vi "CRYCalc Result mean and abs standard.vi"(7 "Step Setup VI No":i32, 8 "Statistic Run Number":i32, 9 "Work in":u16, 11 "Results in":T2 {"Margin" format="%.2f"}) -> (0 "Boolean":bool, 1 "Margin Std Dev Out":T1[](array[typedef]) {"Z data" items=["dB", "Lin"]; "X data" items=["dB", "Lin"]; "Y data" items=["dB", "Lin"]; "Z dB ref" format="%.1f"; "Z axis" items=["Log", "Lin"]; "X dB ref" format="%.1f"; "X axis" items=["Log", "Lin"]; "Y axis" items=["Log", "Lin"]; "Y dB ref" format="%.1f"; "Curve"."z" format="%.2f"; "Curve"."y" format="%.2f"; "Curve"."x" format="%.2f"}, 3 "Margin mean Out":T1[](array[typedef]) {"Z data" items=["dB", "Lin"]; "X data" items=["dB", "Lin"]; "Y data" items=["dB", "Lin"]; "Z dB ref" format="%.1f"; "Z axis" items=["Log", "Lin"]; "X dB ref" format="%.1f"; "X axis" items=["Log", "Lin"]; "Y axis" items=["Log", "Lin"]; "Y dB ref" format="%.1f"; "Curve"."z" format="%.2f"; "Curve"."y" format="%.2f"; "Curve"."x" format="%.2f"})   [LabVIEW 2013]
uses:
  Typedef Control/CRYResult Cluster Array.ctl
  Typedef Control/CRYResult Cluster.ctl
  Typedef Control/CRYData Cluster.ctl
  CRYStatistics Global.vi
  <vilib>/Analysis/NI_AALBase.lvlib
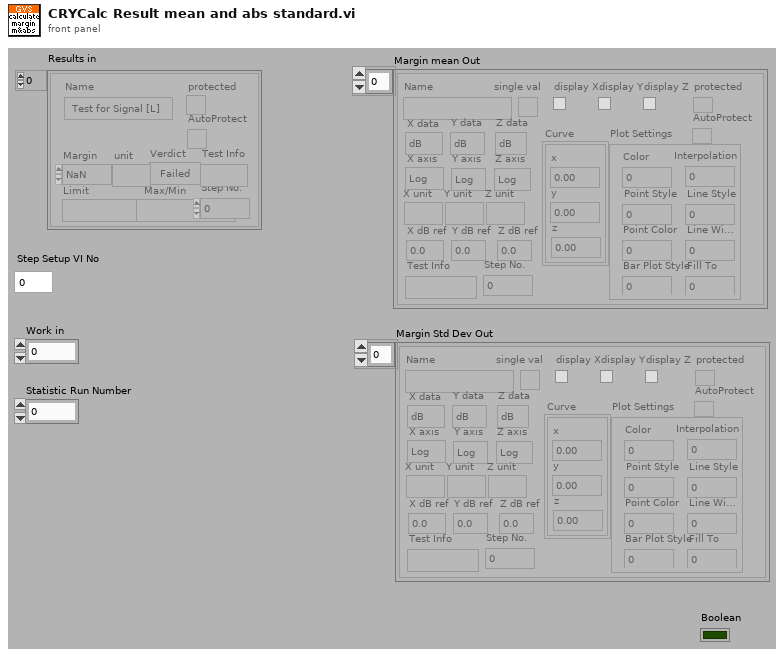
[diagram p1: front panel]
types:
  T1 = typedef "CRYData Cluster.ctl" = cluster{"Name":string, "Curve":cluster{"x":dbl, "y":dbl, "z":dbl}[], "X data":u16, "Y data":u16, "Z data":u16, "X axis":u16, "Y axis":u16, "Z axis":u16, "X unit":string, "Y unit":string, "Z unit":string, "X dB ref":dbl, "Y dB ref":dbl, "Z dB ref":dbl, "single val":bool, "protected":bool, "display X":bool, "display Y":bool, "display Z":bool, "Test Info":string, "Step No.":i32, "Plot Settings":cluster{"Color":u32, "Interpolation":u8, "Point Style":u8, "Line Style":u8, "Point Color":u32, "Line Width":u8, "Bar Plot Style":u8, "Fill To":i16}, "AutoProtect":bool}
  T2 = typedef "CRYResult Cluster Array.ctl" = T3[]
  T3 = typedef "CRYResult Cluster.ctl" = cluster{"Name":string, "Margin":dbl, "unit":string, "Verdict":bool, "Limit":string, "Max/Min":string, "protected":bool, "Step No.":i32, "Test Info":string, "AutoProtect":bool}
  T4 = enum32{"English", "Chinese", "Korean", "Japanese", "Russian", "Chinese traditional"}
  T5 = typedef "CRYData Cluster Array.ctl" = T1[]
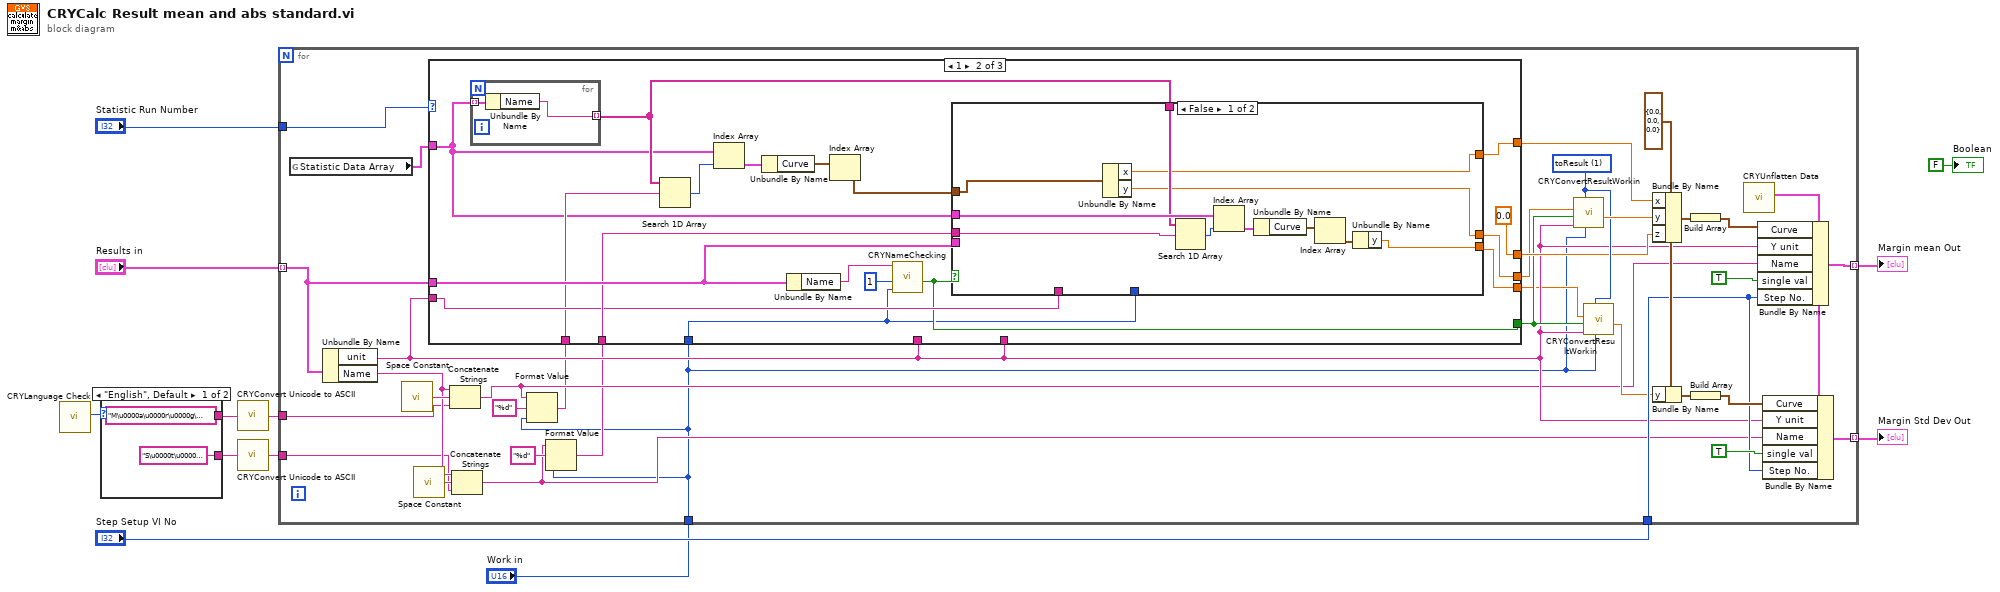
[diagram p0: block diagram]
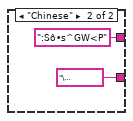
[diagram p2: hidden frame]
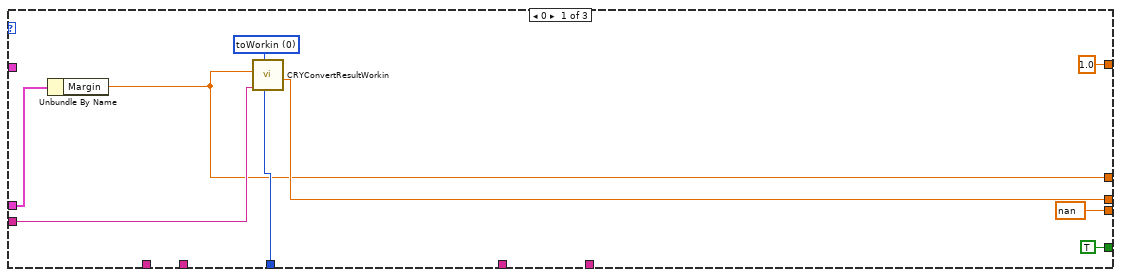
[diagram p3: hidden frame]
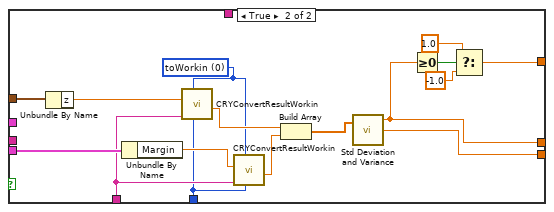
[diagram p4: hidden frame]
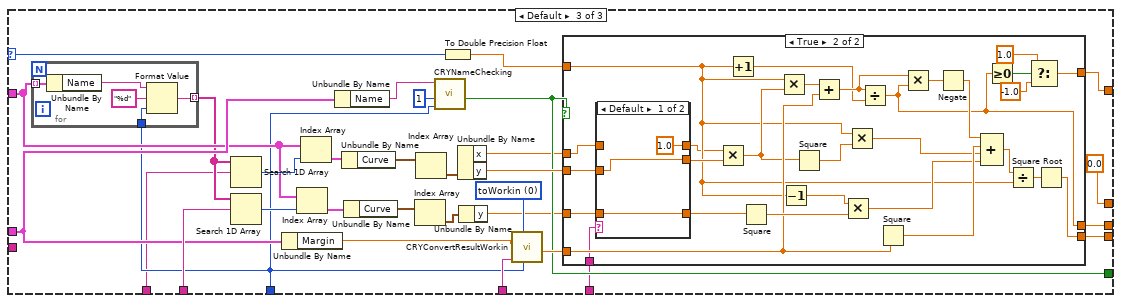
[diagram p5: hidden frame]
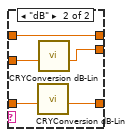
[diagram p7: hidden frame]
diagram:
  n1 = call "CRYLanguage Check.vi"() -> ("Language"=w5:T4)  [unwired: 10 in, 1 out]
  n2 = case shown="\"English\", Default" w5 {
    tunnel: ["M\u0000a\u0000r\u0000g\u0000i\u0000n\u0000 \u0000M\u0000e\u0000a\u0000n\u0000" ("format string") ":Sô•s^GW<P" ("format string")] -> w6
    tunnel: ["S\u0000t\u0000d\u0000 \u0000D\u0000e\u0000v\u0000" ("format string") "\u0007hÆQî]" ("format string")] -> w4
    frame "English", Default {
    }
    frame "Chinese" {
    }
  }
  n3 = call "CRYConvert Unicode to ASCII.vi"("Unicode"=w6) -> ("ASCII"=w3:string)  [unwired: 4 in]
  n4 = call "CRYConvert Unicode to ASCII.vi"("Unicode"=w4) -> ("ASCII"=w2:string)  [unwired: 4 in]
  n5 = for {
    tunnel: "Results in" -> [w33] mode=indexing
    tunnel: [w48] -> w11 mode=indexing
    tunnel: [w42] -> w10 mode=indexing
    tunnel: "Step Setup VI No" -> [w41]
    tunnel: "Statistic Run Number" -> [w40]
    tunnel: w3 -> [w35]
    tunnel: w2 -> [w34]
    tunnel: "Work in" -> [w17]
    w31 = u16 1 items=["toWorkin", "toResult"] ("Type")
    w43 = cluster{"x":dbl, "y":dbl, "z":dbl} {"x"=0.0, "y"=0.0, "z"=0.0}
    n6 = global read "CRYStatistics Global.vi" "Statistic Data Array"() -> (w36:T5)
    n7 = Unbundle By Name(w33) -> ("unit"=w27:string, "Name"=w37:string)
    n8 = call <vilib>:"Space Constant.vi"() -> ("String"=w39:string)
    n9 = call <vilib>:"Space Constant.vi"() -> ("String"=w38:string)
    n10 = Concatenate Strings(w37, w39, w35) -> (w22:string)
    n11 = Concatenate Strings(w37, w38, w34) -> (w19:string)
    n12 = Format Value(string ("")=w22, format string="%d", value (0)=w17) -> (output string=w21:string)
    n13 = Format Value(string ("")=w19, format string="%d", value (0)=w17) -> (output string=w18:string)
    n14 = case shown="1" w40 {
      selector: w40 -> [_ _ w117]
      tunnel: w33 -> [w59 w73 w124]
      tunnel: w18 -> [_ w70 w137]
      tunnel: [w57 w75 w129] -> w26
      tunnel: [nan ("y") w74 w128] -> w25
      tunnel: w36 -> [_ w62 w111]
      tunnel: w27 -> [w60 w69 _]
      tunnel: w17 -> [w55 w61 w109]
      tunnel: w27 -> [_ _ w123]
      tunnel: [w54 0.0 ("Margin") 0.0 ("Margin")] -> w29
      tunnel: [TRUE ("Out Calcurated") w66 w116] -> w28
      tunnel: w27 -> [_ _ w115]
      tunnel: [1.0 ("f") w65 w113] -> w24
      tunnel: w21 -> [_ w64 w108]
      frame 0 {
        w58 = u16 0 items=["toWorkin", "toResult"] ("Type")
        n15 = Unbundle By Name(w59) -> ("Margin"=w54:dbl)
        n16 = call "CRYConvertResultWorkin.vi"("Work in"=w55, "Type"=w58, "unit"=w60, "Margin In"=w54) -> ("Margin Out"=w57:dbl)  [unwired: 7 in]
      }
      frame 1 {
        n17 = for {
          tunnel: w62 -> [w80] mode=indexing
          tunnel: [w79] -> w63 mode=indexing
          n18 = Unbundle By Name(w80) -> ("Name"=w79:string)
        }
        n19 = Search 1D Array(1D array=w63, element=w64) -> (index of element=w78:i32)  [unwired: 1 in]
        n20 = Index Array(array=w62, index=w78) -> (element=w77:T1)
        n21 = Unbundle By Name(w77) -> ("Curve"=w76:cluster{"x":dbl, "y":dbl, "z":dbl}[])
        n22 = Unbundle By Name(w73) -> ("Name"=w72:string)
        n23 = Index Array(array=w76) -> (element=w67:cluster{"x":dbl, "y":dbl, "z":dbl})  [unwired: 1 in]
        n24 = call "CRYNameChecking.vi"("Curve Name"=w72, "Mode"=i8 1, "Work in"=w61) -> ("Out Calcurated"=w66:bool)  [unwired: 7 in]
        n25 = case shown="False" w66 {
          tunnel: w67 -> [w84 w99]
          tunnel: [w83 w94] -> w75
          tunnel: [w82 w92] -> w74
          tunnel: w73 -> [_ w106]
          tunnel: w70 -> [w87 _]
          tunnel: w62 -> [w86 _]
          tunnel: w63 -> [w85 _]
          tunnel: w69 -> [_ w103]
          tunnel: w61 -> [_ w102]
          tunnel: [w81 w93] -> w65
          frame False {
            n26 = Unbundle By Name(w84) -> ("x"=w81:dbl, "y"=w83:dbl)
            n27 = Search 1D Array(1D array=w85, element=w87) -> (index of element=w88:i32)  [unwired: 1 in]
            n28 = Index Array(array=w86, index=w88) -> (element=w89:T1)
            n29 = Unbundle By Name(w89) -> ("Curve"=w90:cluster{"x":dbl, "y":dbl, "z":dbl}[])
            n30 = Index Array(array=w90) -> (element=w91:cluster{"x":dbl, "y":dbl, "z":dbl})  [unwired: 1 in]
            n31 = Unbundle By Name(w91) -> ("y"=w82:dbl)
          }
          frame True {
            w101 = u16 0 items=["toWorkin", "toResult"] ("Type")
            n32 = Unbundle By Name(w99) -> ("z"=w98:dbl)
            n33 = Unbundle By Name(w106) -> ("Margin"=w104:dbl)
            n34 = call "CRYConvertResultWorkin.vi"("Work in"=w102, "Type"=w101, "unit"=w103, "Margin In"=w98) -> ("Margin Out"=w105:dbl)  [unwired: 7 in]
            n35 = call "CRYConvertResultWorkin.vi"("Work in"=w102, "Type"=w101, "unit"=w103, "Margin In"=w104) -> ("Margin Out"=w100:dbl)  [unwired: 7 in]
            n36 = Build Array(w105, w100) -> (w107:dbl[])
            n37 = call <vilib>:"Std Deviation and Variance.vi"("X"=w107) -> ("mean"=w94:dbl, "standard deviation"=w92:dbl)  [unwired: 1 in, 1 out]
            n38 = Greater Or Equal To 0?(x=w94) -> (x >= 0?=w95:bool)
            n39 = Select(t=1.0, s=w95, f=-1.0) -> (s? t:f=w93:dbl)
          }
        }
      }
      frame Default {
        w118 = u16 0 items=["toWorkin", "toResult"] ("Type")
        n40 = for {
          tunnel: w111 -> [w143] mode=indexing
          tunnel: w109 -> [w140]
          tunnel: [w139] -> w110 mode=indexing
          n41 = Unbundle By Name(w143) -> ("Name"=w141:string)
          n42 = Format Value(string ("")=w141, format string="%d", value (0)=w140) -> (output string=w139:string)
        }
        n43 = Search 1D Array(1D array=w110, element=w108) -> (index of element=w138:i32)  [unwired: 1 in]
        n44 = Search 1D Array(1D array=w110, element=w137) -> (index of element=w136:i32)  [unwired: 1 in]
        n45 = Unbundle By Name(w124) -> ("Margin"=w122:dbl)
        n46 = Index Array(array=w111, index=w136) -> (element=w134:T1)
        n47 = Index Array(array=w111, index=w138) -> (element=w135:T1)
        n48 = Unbundle By Name(w124) -> ("Name"=w125:string)
        n49 = Unbundle By Name(w135) -> ("Curve"=w133:cluster{"x":dbl, "y":dbl, "z":dbl}[])
        n50 = Unbundle By Name(w134) -> ("Curve"=w132:cluster{"x":dbl, "y":dbl, "z":dbl}[])
        n51 = Index Array(array=w132) -> (element=w130:cluster{"x":dbl, "y":dbl, "z":dbl})  [unwired: 1 in]
        n52 = Index Array(array=w133) -> (element=w131:cluster{"x":dbl, "y":dbl, "z":dbl})  [unwired: 1 in]
        n53 = call "CRYNameChecking.vi"("Curve Name"=w125, "Mode"=i8 1, "Work in"=w109) -> ("Out Calcurated"=w116:bool)  [unwired: 7 in]
        n54 = To Double Precision Float(number=w117) -> (double precision float=w127:dbl)
        n55 = Unbundle By Name(w131) -> ("x"=w114:dbl, "y"=w119:dbl)
        n56 = Unbundle By Name(w130) -> ("y"=w112:dbl)
        n57 = call "CRYConvertResultWorkin.vi"("Work in"=w109, "Type"=w118, "unit"=w123, "Margin In"=w122) -> ("Margin Out"=w121:dbl)  [unwired: 7 in]
        n58 = case shown="True" w116 {
          tunnel: w121 -> [_ w164]
          tunnel: w119 -> [w145 w159]
          tunnel: w112 -> [w146 w161]
          tunnel: [w145 w153] -> w129
          tunnel: [w146 w151] -> w128
          tunnel: w127 -> [_ w148]
          tunnel: w115 -> [_ w158]
          tunnel: w114 -> [w144 w149]
          tunnel: [w144 w152] -> w113
          frame False {
          }
          frame True {
            n59 = case shown="Default" w158 {
              tunnel: w161 -> [w177 w183]
              tunnel: [w177 w182] -> w160
              tunnel: w159 -> [w178 w181]
              tunnel: [w178 w180] -> w157
              tunnel: [1.0 ("x") w179] -> w147
              tunnel: w149 -> [_ w179]
              frame Default {
              }
              frame "dB" {
                n60 = call "CRYConversion dB-Lin.vi"("Log In"=w183) -> ("Lin Out"=w182:dbl)  [unwired: 5 in, 3 out]
                n61 = call "CRYConversion dB-Lin.vi"("Log In"=w181) -> ("Lin Out"=w180:dbl)  [unwired: 5 in, 3 out]
              }
            }
            n62 = Multiply(x=w147, y=w157) -> (x*y=w156:dbl)
            n63 = Increment(x=w148) -> (x+1=w163:dbl)
            n64 = Square(x=w160) -> (x^2=w174:dbl)
            n65 = Multiply(x=w148, y=w156) -> (x*y=w175:dbl)
            n66 = Decrement(x=w148) -> (x-1=w162:dbl)
            n67 = Square(x=w156) -> (x^2=w173:dbl)
            n68 = Add(x=w175, y=w164) -> (x+y=w169:dbl)
            n69 = Multiply(x=w162, y=w174) -> (x*y=w170:dbl)
            n70 = Multiply(x=w148, y=w173) -> (x*y=w171:dbl)
            n71 = Divide(x=w169, y=w163) -> (x/y=w153:dbl)
            n72 = Square(x=w164) -> (x^2=w172:dbl)
            n73 = Multiply(x=w169, y=w153) -> (x*y=w168:dbl)
            n74 = Negate(x=w168) -> (-x=w167:dbl)
            n75 = Compound Arithmetic op=ADD(w167, w172, w171, w170) -> (w166:dbl)
            n76 = Greater Or Equal To 0?(x=w153) -> (x >= 0?=w155:bool)
            n77 = Divide(x=w166, y=w148) -> (x/y=w165:dbl)
            n78 = Select(t=1.0, s=w155, f=-1.0) -> (s? t:f=w152:dbl)
            n79 = Square Root(x=w165) -> (sqrt(x)=w151:dbl)
          }
        }
      }
    }
    n80 = call "CRYConvertResultWorkin.vi"("Work in"=w17, "Type"=w31, "unit"=w27, "IsTrue"=w28, "Margin In"=w26) -> ("Margin Out"=w32:dbl)  [unwired: 6 in]
    n81 = call "CRYConvertResultWorkin.vi"("Work in"=w17, "Type"=w31, "unit"=w27, "IsTrue"=w28, "Margin In"=w25) -> ("Margin Out"=w30:dbl)  [unwired: 6 in]
    n82 = Bundle By Name(cluster=w43, "x"=w24, "y"=w32, "z"=w29) -> (w51:cluster{"x":dbl, "y":dbl, "z":dbl})
    n83 = Bundle By Name(cluster=w43, "y"=w30) -> (w45:cluster{"x":dbl, "y":dbl, "z":dbl})
    n84 = Build Array(w51) -> (w49:cluster{"x":dbl, "y":dbl, "z":dbl}[])
    n85 = Build Array(w45) -> (w47:cluster{"x":dbl, "y":dbl, "z":dbl}[])
    n86 = call "CRYUnflatten Data.vi"() -> ("Datum"=w44:T1)  [unwired: 9 in, 2 out]
    n87 = Bundle By Name(cluster=w44, "Curve"=w49, "Y unit"=w27, "Name"=w22, "single val"=TRUE, "Step No."=w41) -> (w48:T1)
    n88 = Bundle By Name(cluster=w44, "Curve"=w47, "Y unit"=w27, "Name"=w19, "single val"=TRUE, "Step No."=w41) -> (w42:T1)
  }
  "Margin mean Out" <- w11
  "Margin Std Dev Out" <- w10
  "Boolean" <- FALSE ("Boolean")
